vi "Create default Layer.vi"(8 "error in (no error)":errorcluster) -> (0 "error out":errorcluster, 3 "Layer.lvclass out":refnum<class "Layer.lvclass">)   [LabVIEW 2020, in "lv_icon.lvlib"]
doc: "Create a default User Layer.\nBlack rectangle border.\n100% Opacity\nEmpty Layer Name"
uses:
  lv_icon.lvlib
  Classes/Layer/Layer.lvclass
  Controls/Layer.ctl
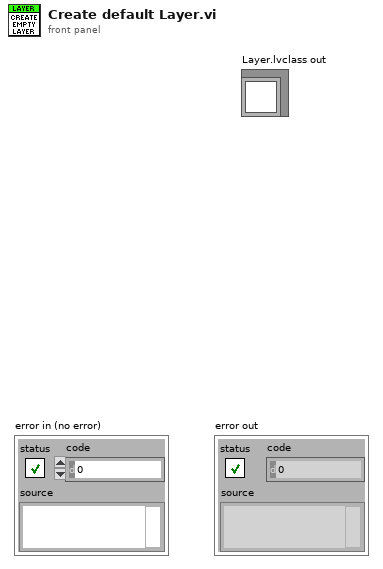
[diagram p1: front panel]
types:
  T1 = typedef "Layer.ctl" = cluster{"LayerIcon":picture, "LayerName":string, "Opacity":u8, "Visibility?":bool}
  T2 = cluster{"left":i16, "top":i16, "right":i16, "bottom":i16}
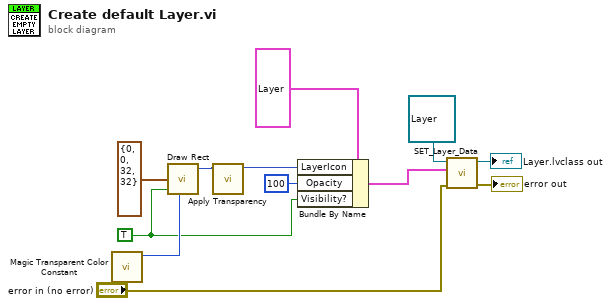
[diagram p0: block diagram]
diagram:
  w1 = TRUE ("fill?(F)")
  n1 = call "Magic Transparent Color Constant.vi"() -> ("Magic transparent color constant"=w5:u32)  [unwired: 11 out]
  n2 = call <vilib>:"Draw Rect.vi"("rect"=T2 {"left"=0, "top"=0, "right"=32, "bottom"=32}, "fill?(F)"=w1, "color(black)"=w5) -> ("new picture"=w3:picture)  [unwired: 2 in, 4 out]
  n3 = call "Apply Transparency.vi"("in"=w3) -> ("out"=w4:picture)  [unwired: 1 in, 9 out]
  n4 = Bundle By Name(cluster=T1 {"LayerIcon"=bytes[0], "LayerName"="", "Opacity"=0, "Visibility?"=FALSE} ("Data"), "LayerIcon"=w4, "Opacity"=u8 100, "Visibility?"=w1) -> (w10:T1)
  n5 = call-dynamic "SET_Layer_Data.vi"("error in (no error)"="error in (no error)", "Data"=w10, "Layer.lvclass in"=refnum<class "Layer.lvclass"> refnum) -> ("error out"=→"error out":errorcluster, "Layer.lvclass out"=→"Layer.lvclass out":refnum<class "Layer.lvclass">)  [unwired: 1 in, 6 out]
